vi "Write class.vi"(8 "error in (no error)":errorcluster, 10 "class":string, 11 "Element in":refnum<class "Element.lvclass">) -> (0 "error out":errorcluster, 3 "Element out":refnum<class "Element.lvclass">)   [LabVIEW 2020, in "VILab.lvlib" / "Element.lvclass"]
uses:
  Element.lvclass
  Element.lvclass/Element.ctl
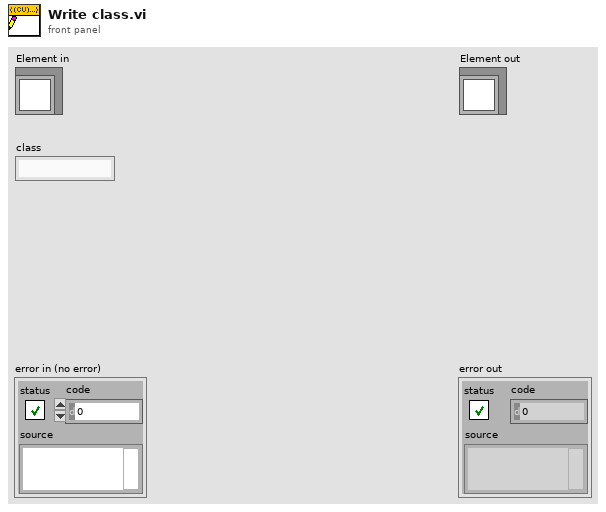
[diagram p1: front panel]
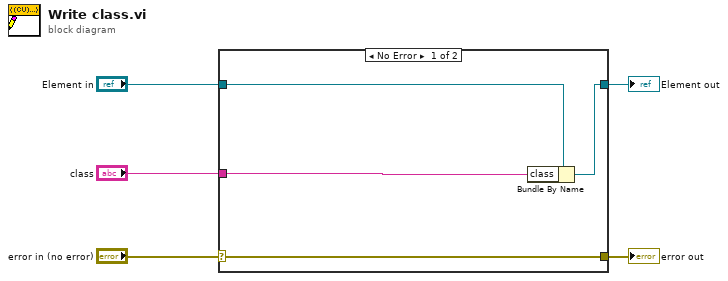
[diagram p0: block diagram]
diagram:
  n1 = case shown="No Error" "error in (no error)" {
    selector: "error in (no error)" -> [w9 w10]
    tunnel: [w9 w10] -> w4
    tunnel: [w7 w11] -> w2
    tunnel: "Element in" -> [w8 w11]
    tunnel: "class" -> [w6 _]
    frame No Error {
      n2 = Bundle By Name(cluster=w8, "class"=w6) -> (w7:refnum<class "Element.lvclass">)
    }
    frame Error {
    }
  }
  "error out" <- w4
  "Element out" <- w2
